vi "LVClass_HasoField Read Haso Field ptr create.vi"(8 "error in (no error)":errorcluster, 11 "HasoField in":refnum<class "HasoField.lvclass">) -> (0 "error out":errorcluster, 2 "Enum":T1, 3 "HasoField out":refnum<class "HasoField.lvclass">)   [LabVIEW 2020, in "HasoField.lvclass"]
uses:
  HasoField.lvclass
  Controls/Handle creation.ctl
  HasoField.lvclass/HasoField.ctl
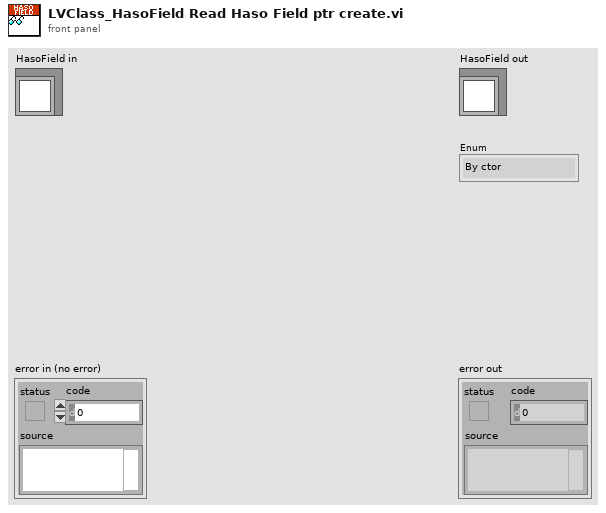
[diagram p1: front panel]
types:
  T1 = typedef "Handle creation.ctl" = enum16{"By ctor", "By write function"}
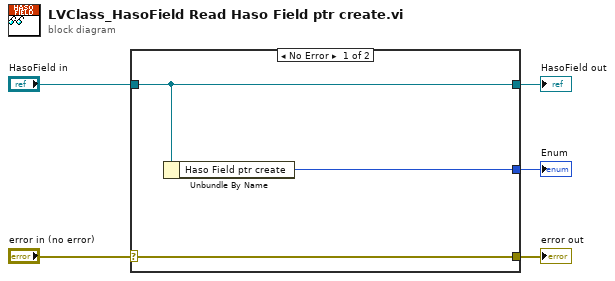
[diagram p0: block diagram]
diagram:
  n1 = case shown="No Error" "error in (no error)" {
    selector: "error in (no error)" -> [w8 w9]
    tunnel: [w8 w9] -> w4
    tunnel: [w7 w10] -> w2
    tunnel: "HasoField in" -> [w7 w10]
    tunnel: [w6 _] -> w1
    frame No Error {
      n2 = Unbundle By Name(w7) -> ("Haso Field ptr create"=w6:T1)
    }
    frame Error {
    }
  }
  "error out" <- w4
  "HasoField out" <- w2
  "Enum" <- w1
